vi "Stack-Statistics.vi"(4 "Theshold":dbl=100.0, 6 "offset":dbl=3200.0, 7 "Enum":T1(ring), 11 "16-bit pixmap":u16[][][](array[numeric])) -> (3 "Out":u16[][](graph))   [LabVIEW 2011]
uses:
  <vilib>/Analysis/NI_AALBase.lvlib
panel:
  out "size(s) 2":i32[](array[numeric])
  out "size(s)":i32[](array[numeric])
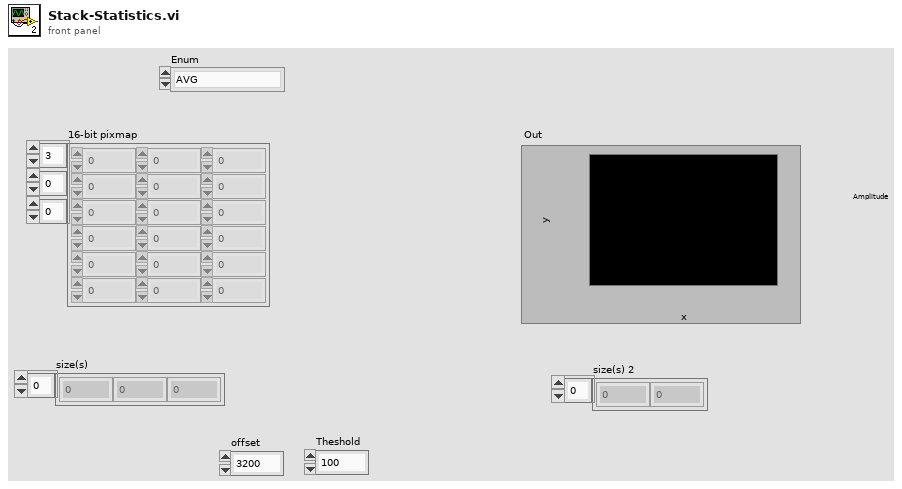
[diagram p1: front panel]
types:
  T1 = enum16{"AVG", "STD", "Contrast1000", "Max", "Min", ""}
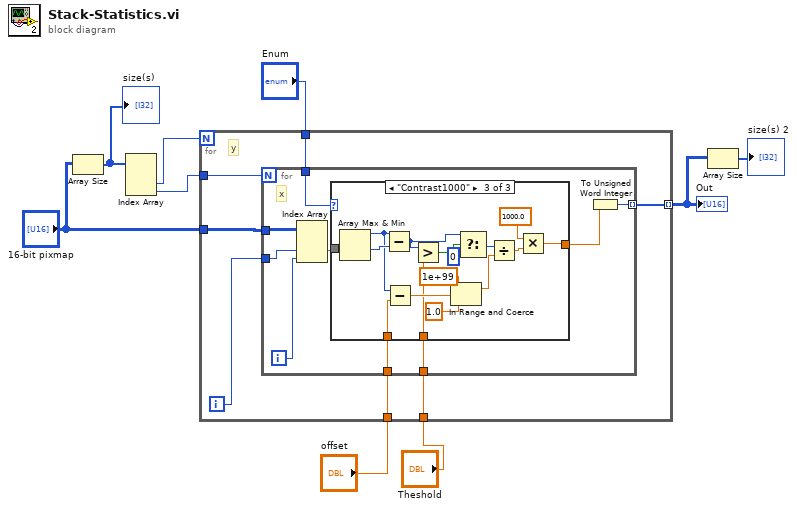
[diagram p0: block diagram]
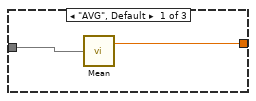
[diagram p2: hidden frame]
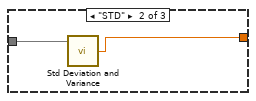
[diagram p3: hidden frame]
diagram:
  n1 = Array Size(array="16-bit pixmap") -> (size(s)=w9:i32[])
  "size(s)" <- w9
  n2 = Index Array(array=w9) -> (element #2=w5:i32, element #3=w6:i32)  [unwired: 3 in, 1 out]
  n3 = for {
    N: w5 -> [_]
    tunnel: "16-bit pixmap" -> [w16]
    tunnel: "Enum" -> [w15]
    tunnel: w6 -> [w14]
    tunnel: [w12] -> w4 mode=indexing
    tunnel: "offset" -> [w11]
    tunnel: "Theshold" -> [w10]
    i -> [w13]
    # "y"
    n4 = for {
      N: w14 -> [_]
      tunnel: w16 -> [w25]
      tunnel: w15 -> [w23]
      tunnel: w13 -> [w19]
      tunnel: [w21] -> w12 mode=indexing
      tunnel: w11 -> [w18]
      tunnel: w10 -> [w17]
      i -> [w20]
      # "x"
      n5 = Index Array(array=w25, index (dim 1)=w19, index (dim 2)=w20) -> (element=w24:u16[])  [unwired: 1 in]
      n6 = case shown="\"Contrast1000\"" w23 {
        tunnel: w24 -> [w27 w29 w45]
        tunnel: [w26 w28 w40] -> w22
        tunnel: w18 -> [_ _ w43]
        tunnel: w17 -> [_ _ w34]
        frame "AVG", Default {
          n7 = call <vilib>:"Mean.vi"("X"=w27) -> ("mean"=w26:dbl)  [unwired: 1 out]
        }
        frame "STD" {
          n8 = call <vilib>:"Std Deviation and Variance.vi"("X"=w29) -> ("standard deviation"=w28:dbl)  [unwired: 1 in, 2 out]
        }
        frame "Contrast1000" {
          n9 = Array Max & Min(array=w45) -> (max value=w30:u16, min value=w44:u16)  [unwired: 2 out]
          n10 = Subtract(x=w30, y=w44) -> (x-y=w35:u16)
          n11 = Subtract(x=w30, y=w43) -> (x-y=w39:dbl)
          n12 = Greater?(x=w35, y=w34) -> (0:w32:bool)
          n13 = In Range and Coerce(upper limit=1e+99, x=w39, lower limit=1.0) -> (coerced(x)=w37:dbl)  [unwired: 1 out]
          n14 = Select(t=w35, s=w32, f=u16 0) -> (s? t:f=w33:u16)
          n15 = Divide(x=w33, y=w37) -> (x/y=w42:dbl)
          n16 = Multiply(x=1000.0, y=w42) -> (x*y=w40:dbl)
        }
      }
      n17 = To Unsigned Word Integer(number=w22) -> (unsigned 16bit integer=w21:u16)
    }
  }
  "Out" <- w4
  n18 = Array Size(array=w4) -> (size(s)=→"size(s) 2":i32[])
